vi "SVXMPL_Override DAQ Parameters.vi"(0 "acquisition task in":T4={"AI device settings"={"AI device"=1, "AI taskID"=0, "response"=[]}, "acquisition type"=enum."Finite", "measurement settings"={"AI sampling frequency"=51200.0, "AO sampling frequency"=51200.0, "AI block size"=1024, "AO block Size"=0, "block duration [ms]"=1024.0, "number of AI channels"=0, "board propagation time [samples]"=0, "DUT propagation time [s]"=0.0}, "settling settings"={"settle time"=0.015599999576807022, "settle cycles"=5}, "integration settings"={"integration time"=0.015599999576807022, "integration cycles"=5}, "AO device settings"={"AO device"=1, "AO taskID"=0, "excitation"=[]}, "acquisition accounting"={"initial read size [samples]"=0, "read offset [samples]"=0, "read length [samples]"=0, "blocks to settle [samples]"=0, "min delay until transition [samples]"=0}, "frequency range"={"start frequency"=0.015599999576807022, "stop frequency"=5.0}, "block type"=enum."Initialize", "source settings"={"signal type"=enum."Dual tone (IMD)", "frequency"=0.0, "total amplitude"=0.0, "frequencies"=[1.0], "relative amplitudes"=[1.0], "offset"=1.0, "total amplitude list"=[1.0], "ramping rate"=0.0}} {"source settings"."total amplitude" format="%.2f"; "source settings"."relative amplitudes" format="%.2f"; "source settings"."frequencies" format="%.2f"; "source settings"."total amplitude list" format="%.2f"; "source settings"."ramping rate" format="%.4f"; "source settings"."offset" format="%.2f"; "source settings"."frequency" format="%.2f"; "frequency range"."stop frequency" format="%.2f"; "frequency range"."start frequency" format="%.2f"; "AO device settings"."excitation"."output limits"."low limit (-10 V)" format="%.2f"; "AO device settings"."excitation"."output limits"."high limit (10 V)" format="%.2f"; "AI device settings"."response"."input limits"."low limit (0.0)" format="%.2f"; "AI device settings"."response"."input limits"."high limit (0.0)" format="%.2f"; "integration settings"."integration time" format="%.2p"; "settling settings"."settle time" format="%.2p"; "measurement settings"."DUT propagation time [s]" format="%.2f"; "measurement settings"."AO sampling frequency" format="%.2f"; "measurement settings"."AI sampling frequency" format="%.2f"}, 1 "output limits\n(empty: no change)":T1(array[cluster]) {"low limit (-10 V)" format="%.2f"; "high limit (10 V)" format="%.2f"}, 2 "input limits\n(empty: no change)":T3(array[cluster]) {"low limit (0.0)" format="%.2f"; "high limit (0.0)" format="%.2f"}, 3 "coupling & input config\n(empty: no change)":T2(array[cluster]), 5 "block size\n(-1: no change)":i32=-1, 7 "sampling frequency\n(-1: no change)":dbl=-1.0 format="%.2f", 11 "error in (no error)":errorcluster, 12 "enable manual override (T)":bool=TRUE) -> (4 "acquisition task out":T4={"AI device settings"={"AI device"=1, "AI taskID"=0, "response"=[]}, "acquisition type"=enum."Finite", "measurement settings"={"AI sampling frequency"=51200.0, "AO sampling frequency"=51200.0, "AI block size"=1024, "AO block Size"=0, "block duration [ms]"=1024.0, "number of AI channels"=0, "board propagation time [samples]"=0, "DUT propagation time [s]"=0.0}, "settling settings"={"settle time"=0.015599999576807022, "settle cycles"=5}, "integration settings"={"integration time"=0.015599999576807022, "integration cycles"=5}, "AO device settings"={"AO device"=1, "AO taskID"=0, "excitation"=[]}, "acquisition accounting"={"initial read size [samples]"=0, "read offset [samples]"=0, "read length [samples]"=0, "blocks to settle [samples]"=0, "min delay until transition [samples]"=0}, "frequency range"={"start frequency"=0.015599999576807022, "stop frequency"=5.0}, "block type"=enum."Initialize", "source settings"={"signal type"=enum."Dual tone (IMD)", "frequency"=0.0, "total amplitude"=0.0, "frequencies"=[1.0], "relative amplitudes"=[1.0], "offset"=1.0, "total amplitude list"=[1.0], "ramping rate"=0.0}} {"source settings"."total amplitude" format="%.2f"; "source settings"."relative amplitudes" format="%.2f"; "source settings"."frequencies" format="%.2f"; "source settings"."total amplitude list" format="%.2f"; "source settings"."ramping rate" format="%.4f"; "source settings"."offset" format="%.2f"; "source settings"."frequency" format="%.2f"; "frequency range"."stop frequency" format="%.2f"; "frequency range"."start frequency" format="%.2f"; "AO device settings"."excitation"."output limits"."low limit (-10 V)" format="%.2f"; "AO device settings"."excitation"."output limits"."high limit (10 V)" format="%.2f"; "AI device settings"."response"."input limits"."low limit (0.0)" format="%.2f"; "AI device settings"."response"."input limits"."high limit (0.0)" format="%.2f"; "integration settings"."integration time" format="%.2p"; "settling settings"."settle time" format="%.2p"; "measurement settings"."DUT propagation time [s]" format="%.2f"; "measurement settings"."AO sampling frequency" format="%.2f"; "measurement settings"."AI sampling frequency" format="%.2f"}, 15 "error out":errorcluster)   [LabVIEW 2017]
doc: "This example VI allows you to overwrite specific data-acquisition parameters for a synchronzed AO/AI measurement.\n\nIf you want to leave this VI in the data flow, but disallow manual overwrites, set <B>enable manual override</B> to FALSE.\n\nYou can change any of the supported DAQ parameters to customize this example to your needs, and you can choose to leave the DAQ parameters at their automatic values by leaving the inputs to this VI at their default values."
uses:
  <vilib>/addons/Sound and Vibration/compatibility/Example Support/SVXMPL_Acquisition Task.ctl
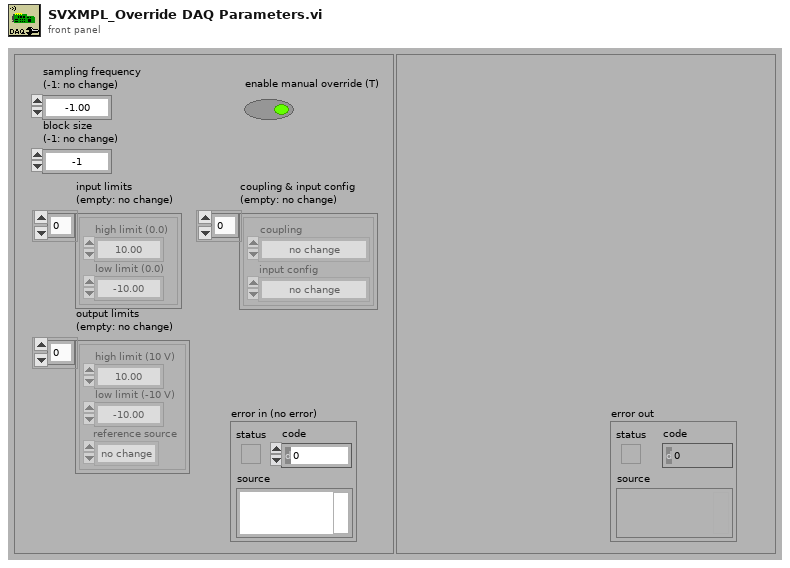
[diagram p1: front panel]
types:
  T1 = cluster{"high limit (10 V)":sgl, "low limit (-10 V)":sgl, "reference source":enum16{"no change", "internal", "external"}}[]
  T2 = cluster{"coupling":enum16{"no change", "DC", "AC", "GND", "internal ref."}, "input config":enum16{"no change", "differential", "ref. single-ended", "non-ref. single-ended", "4-wire"}}[]
  T3 = cluster{"high limit (0.0)":sgl, "low limit (0.0)":sgl}[]
  T4 = typedef "SVXMPL_Acquisition Task.ctl" = cluster{"AI device settings":cluster{"AI device":i16, "AI taskID":u32, "response":cluster{"AI channel":tag, "input limits":cluster{"high limit (0.0)":sgl, "low limit (0.0)":sgl}, "coupling & input config":cluster{"coupling":enum16{"no change", "DC", "AC", "GND", "internal ref."}, "input config":enum16{"no change", "differential", "ref. single-ended", "non-ref. single-ended", "4-wire"}}}[]}, "acquisition type":enum16{"Finite", "Averaged", "Settled", "Amplitude Sweep"}, "measurement settings":cluster{"AI sampling frequency":dbl, "AO sampling frequency":dbl, "AI block size":i32, "AO block Size":i32, "block duration [ms]":dbl, "number of AI channels":i32, "board propagation time [samples]":i32, "DUT propagation time [s]":dbl}, "settling settings":cluster{"settle time":dbl, "settle cycles":i32}, "integration settings":cluster{"integration time":dbl, "integration cycles":i32}, "AO device settings":cluster{"AO device":i16, "AO taskID":u32, "excitation":cluster{"AO Channel":tag, "output limits":cluster{"high limit (10 V)":sgl, "low limit (-10 V)":sgl, "reference source":enum16{"no change", "internal", "external"}}}[]}, "acquisition accounting":cluster{"initial read size [samples]":i32, "read offset [samples]":i32, "read length [samples]":i32, "blocks to settle [samples]":i32, "min delay until transition [samples]":i32}, "frequency range":cluster{"start frequency":dbl, "stop frequency":dbl}, "block type":enum16{"Initialize", "Settle", "Integrate"}, "source settings":cluster{"signal type":enum16{"Sine wave", "Dual tone (IMD)", "Multitone", "Chirp", "Frequency flat chirp", "Uniform white noise", "Gaussian white noise", "Pink noise", "PRN"}, "frequency":dbl, "total amplitude":dbl, "frequencies":dbl[], "relative amplitudes":dbl[], "offset":dbl, "total amplitude list":dbl[], "ramping rate":dbl}}
  T5 = cluster{"AI channel":tag, "input limits":cluster{"high limit (0.0)":sgl, "low limit (0.0)":sgl}, "coupling & input config":cluster{"coupling":enum16{"no change", "DC", "AC", "GND", "internal ref."}, "input config":enum16{"no change", "differential", "ref. single-ended", "non-ref. single-ended", "4-wire"}}}[]
  T6 = cluster{"AO Channel":tag, "output limits":cluster{"high limit (10 V)":sgl, "low limit (-10 V)":sgl, "reference source":enum16{"no change", "internal", "external"}}}[]
  T7 = cluster{"AI channel":tag, "input limits":cluster{"high limit (0.0)":sgl, "low limit (0.0)":sgl}, "coupling & input config":cluster{"coupling":enum16{"no change", "DC", "AC", "GND", "internal ref."}, "input config":enum16{"no change", "differential", "ref. single-ended", "non-ref. single-ended", "4-wire"}}}
  T8 = cluster{"AO Channel":tag, "output limits":cluster{"high limit (10 V)":sgl, "low limit (-10 V)":sgl, "reference source":enum16{"no change", "internal", "external"}}}
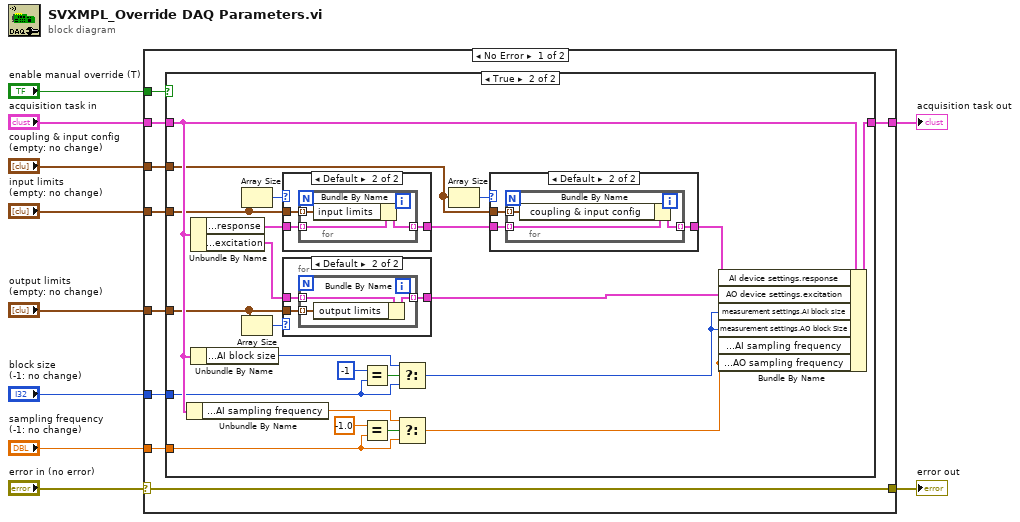
[diagram p0: block diagram]
diagram:
  n1 = case shown="No Error" "error in (no error)" {
    selector: "error in (no error)" -> [w19 w65]
    tunnel: "acquisition task in" -> [w17 w66]
    tunnel: [w18 w66] -> w8
    tunnel: [w19 w65] -> w7
    tunnel: "sampling frequency\n(-1: no change)" -> [w16 _]
    tunnel: "block size\n(-1: no change)" -> [w15 _]
    tunnel: "coupling & input config\n(empty: no change)" -> [w14 _]
    tunnel: "input limits\n(empty: no change)" -> [w13 _]
    tunnel: "output limits\n(empty: no change)" -> [w12 _]
    tunnel: "enable manual override (T)" -> [w11 _]
    frame No Error {
      n2 = case shown="True" w11 {
        tunnel: [w20 w43] -> w18
        tunnel: w17 -> [w20 w37]
        tunnel: w16 -> [_ w31]
        tunnel: w15 -> [_ w30]
        tunnel: w14 -> [_ w21]
        tunnel: w13 -> [_ w25]
        tunnel: w12 -> [_ w26]
        frame False {
        }
        frame True {
          n3 = Unbundle By Name(w37) -> ("measurement settings.AI sampling frequency"=w35:dbl)
          n4 = Unbundle By Name(w37) -> ("AI device settings.response"=w29:T5, "AO device settings.excitation"=w42:T6)
          n5 = Unbundle By Name(w37) -> ("measurement settings.AI block size"=w39:i32)
          n6 = Array Size(array=w25) -> (size(s)=w23:i32)
          n7 = Array Size(array=w26) -> (size(s)=w24:i32)
          n8 = case shown="Default" w23 {
            tunnel: w25 -> [_ w61]
            tunnel: w29 -> [w58 w60]
            tunnel: [w58 w59] -> w28
            frame 0 {
            }
            frame Default {
              n9 = for {
                tunnel: w61 -> [w62] mode=indexing
                tunnel: w60 -> [w64] mode=indexing
                tunnel: [w63] -> w59 mode=indexing
                n10 = Bundle By Name(cluster=w64, "input limits"=w62) -> (w63:T7)
              }
            }
          }
          n11 = case shown="Default" w24 {
            tunnel: w42 -> [w51 w54]
            tunnel: [w51 w53] -> w41
            tunnel: w26 -> [_ w52]
            frame 0 {
            }
            frame Default {
              n12 = for {
                tunnel: w54 -> [w57] mode=indexing
                tunnel: [w56] -> w53 mode=indexing
                tunnel: w52 -> [w55] mode=indexing
                n13 = Bundle By Name(cluster=w57, "output limits"=w55) -> (w56:T8)
              }
            }
          }
          n14 = Equal?(x=-1 ("y"), y=w30) -> (x = y?=w40:bool)
          n15 = Equal?(x=-1.0 ("y"), y=w31) -> (x = y?=w36:bool)
          n16 = Select(t=w39, s=w40, f=w30) -> (s? t:f=w38:i32)
          n17 = Select(t=w35, s=w36, f=w31) -> (s? t:f=w34:dbl)
          n18 = Array Size(array=w21) -> (size(s)=w22:i32)
          n19 = case shown="Default" w22 {
            tunnel: w21 -> [_ w47]
            tunnel: w28 -> [w44 w46]
            tunnel: [w44 w45] -> w27
            frame 0 {
            }
            frame Default {
              n20 = for {
                tunnel: w47 -> [w50] mode=indexing
                tunnel: w46 -> [w49] mode=indexing
                tunnel: [w48] -> w45 mode=indexing
                n21 = Bundle By Name(cluster=w49, "coupling & input config"=w50) -> (w48:T7)
              }
            }
          }
          n22 = Bundle By Name(cluster=w37, "AI device settings.response"=w27, "AO device settings.excitation"=w41, "measurement settings.AI block size"=w38, "measurement settings.AO block Size"=w38, "measurement settings.AI sampling frequency"=w34, "measurement settings.AO sampling frequency"=w34) -> (w43:T4)
        }
      }
    }
    frame Error {
    }
  }
  "acquisition task out" <- w8
  "error out" <- w7
